vi "Voltage Finite Input Wrapper.vi"() -> ()   [LabVIEW 2017]
doc: "This example demonstrates how to acquire a single buffer of voltage measurements using a DAQmx device.\n\nFor instructions on how to connect your signals to the DAQ device, refer to your device documentation."
panel:
  out "String":string
  out "Waveform Graph":waveform(dbl)[](graph)
  in  "TDMS File Path":path
  in  "Logging Mode":i32(ring)=10231 items=["Off"=10231, "Log and Read"=15842]
  # "Channel Settings"
  # "Acquired Data"
  # "Timing Settings"
  # "Trigger Settings"
  # "Logging Settings"
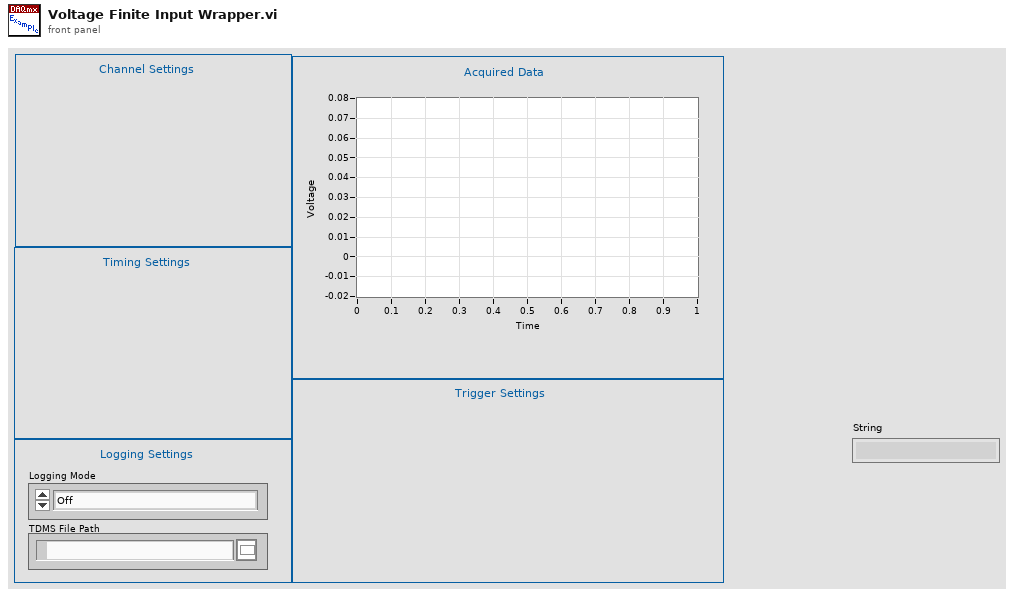
[diagram p1: front panel]
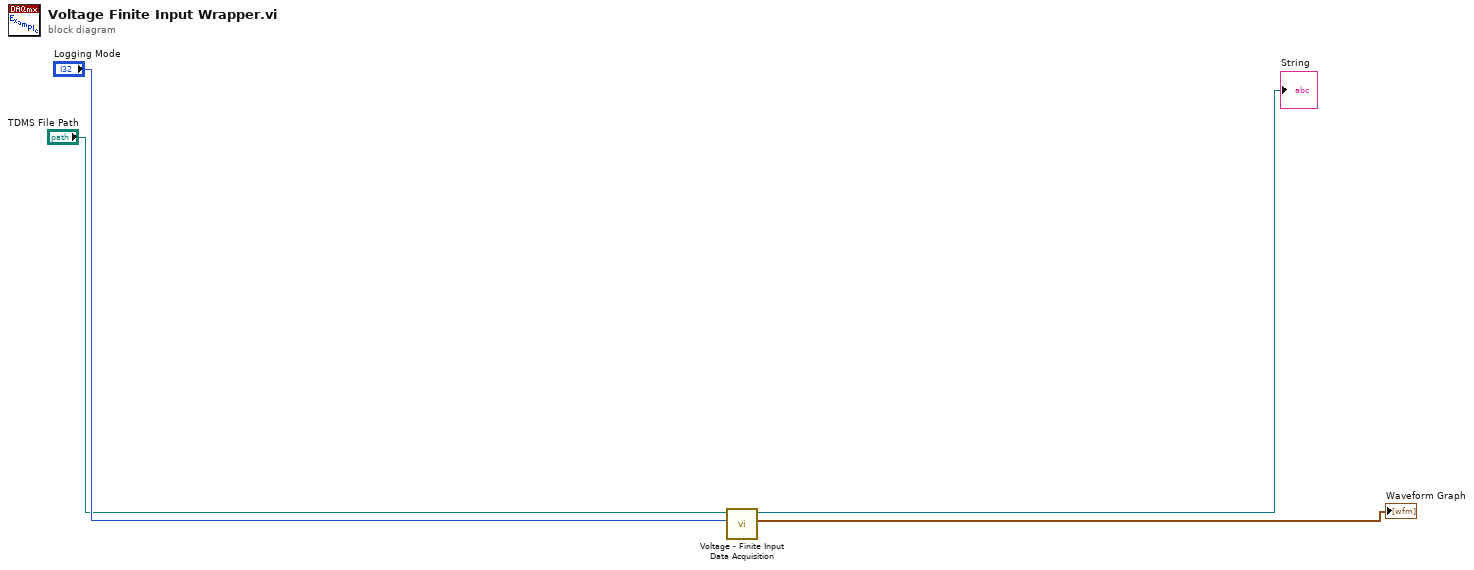
[diagram p0: block diagram]
diagram:
  n1 = call "Voltage - Finite Input Data Acquisition.vi"("Logging Mode"="Logging Mode", "TDMS File Path"="TDMS File Path") -> ("data"=→"Waveform Graph":waveform(dbl)[], "Refnum out"=→"String":refnum<k21>)  [unwired: 8 in]
